vi "Read message.vi"(8 "error in (no error)":errorcluster, 10 "timeout ms (1000)":i32, 11 "WAMP Client in":refnum<class "WAMP Client.lvclass">) -> (0 "error out":errorcluster, 2 "String":string, 3 "WAMP Client out":refnum<class "WAMP Client.lvclass">)   [LabVIEW 2020, in "wamplv.lvlib" / "WAMP Client.lvclass"]
uses:
  WAMP Client.lvclass
  WAMP Client.lvclass/WAMP Client.ctl
  Private/Comm Handlers/ICommHandler/ICommHandler.lvclass
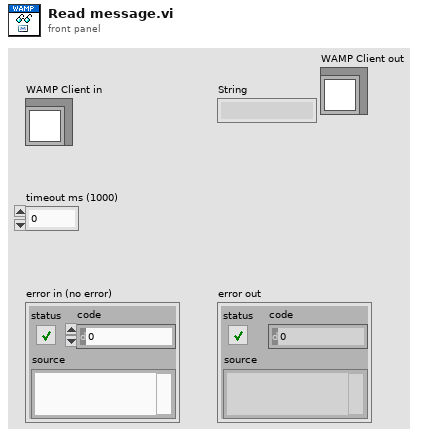
[diagram p1: front panel]
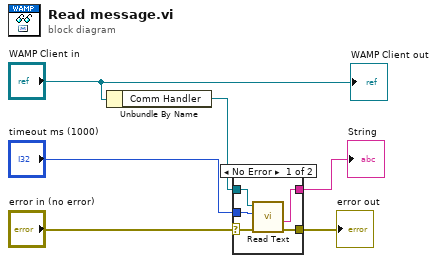
[diagram p0: block diagram]
diagram:
  n1 = Unbundle By Name("WAMP Client in") -> ("Comm Handler"=w5:refnum<class "ICommHandler.lvclass">)
  n2 = case shown="No Error" "error in (no error)" {
    selector: "error in (no error)" -> [w8 w12]
    tunnel: "timeout ms (1000)" -> [w11 _]
    tunnel: w5 -> [w10 _]
    tunnel: [w9 w12] -> w3
    tunnel: [w7 _] -> w1
    frame No Error {
      n3 = call-dynamic "Read Text.vi"("error in (no error)"=w8, "timeout ms (5000)"=w11, "ICommHandler in"=w10) -> ("error out"=w9:errorcluster, "String"=w7:string)  [unwired: 4 in, 1 out]
    }
    frame Error {
    }
  }
  "error out" <- w3
  "String" <- w1
  "WAMP Client out" <- "WAMP Client in"
